vi "ChunkMsg.vi"(8 "Error In":errorcluster, 10 "Input Message":string="Hi, this is Server replying !!!", 11 "SSL Stream":refnum<k24>) -> (0 "Error Out":errorcluster)   [LabVIEW 2014]
uses:
  <userlib>/SSL Library/SSL Lib.lvlib
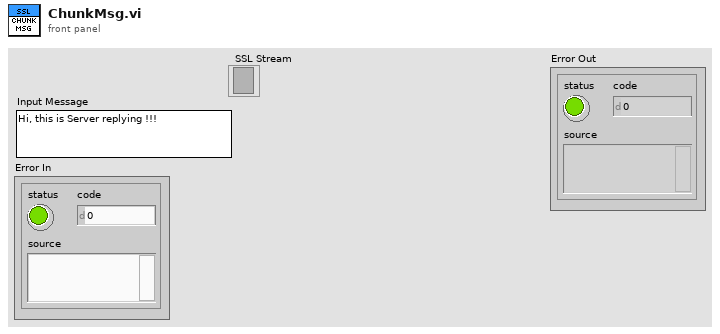
[diagram p1: front panel]
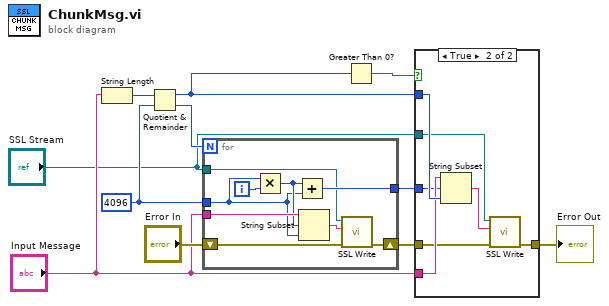
[diagram p0: block diagram]
diagram:
  w9 = 4096 ("y")
  n1 = String Length(string="Input Message") -> (length=w10:i32)
  n2 = Quotient & Remainder(x=w10, y=w9) -> (x-y*floor(x/y)=w6:i32, floor(x/y)=w8:i32)
  n3 = for {
    N: w8 -> [_]
    tunnel: "Input Message" -> [w20]
    shift-right: [w14] -> w2
    shift-left: "Error In" -> [w15]
    tunnel: w9 -> [w17]
    tunnel: [w16] -> w7
    tunnel: "SSL Stream" -> [w13]
    i -> [w19]
    n4 = Multiply(x=w17, y=w19) -> (x*y=w18:i32)
    n5 = Add(x=w18, y=w17) -> (x+y=w16:i32)
    n6 = String Subset(string=w20, offset (0)=w18, length (rest)=w17) -> (substring=w12:string)
    n7 = call "SSL Write.vi"("Error In"=w15, "Input Message"=w12, "SSL Stream"=w13) -> ("Error Out"=w14:errorcluster)  [unwired: 8 in]
  }
  n8 = Greater Than 0?(x=w6) -> (x > 0?=w5:bool)
  n9 = case shown="True" w5 {
    tunnel: w7 -> [_ w26]
    tunnel: w6 -> [_ w28]
    tunnel: "Input Message" -> [_ w27]
    tunnel: [w21 w24] -> w3
    tunnel: w2 -> [w21 w23]
    tunnel: "SSL Stream" -> [_ w22]
    frame False {
    }
    frame True {
      n10 = String Subset(string=w27, offset (0)=w26, length (rest)=w28) -> (substring=w25:string)
      n11 = call "SSL Write.vi"("Error In"=w23, "Input Message"=w25, "SSL Stream"=w22) -> ("Error Out"=w24:errorcluster)  [unwired: 8 in]
    }
  }
  "Error Out" <- w3
